vi "replaceBalanceToken.vi"(8 "error in (no error)":errorcluster, 10 "Query In":string, 11 "Banking Transaction in":refnum<class "Banking Transaction.lvclass">) -> (0 "error out":errorcluster, 2 "Query Out":string, 3 "Banking Transaction out":refnum<class "Banking Transaction.lvclass">)   [LabVIEW 2018, in "Banking Transaction.lvclass"]
uses:
  Banking Transaction.lvclass
  Banking Transaction.lvclass/Banking Transaction.ctl
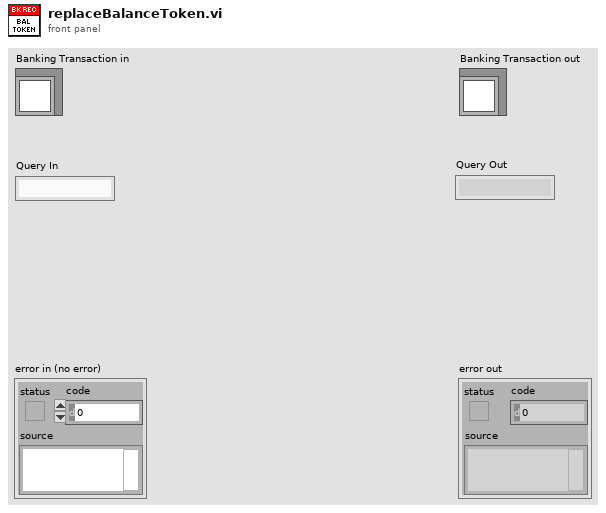
[diagram p1: front panel]
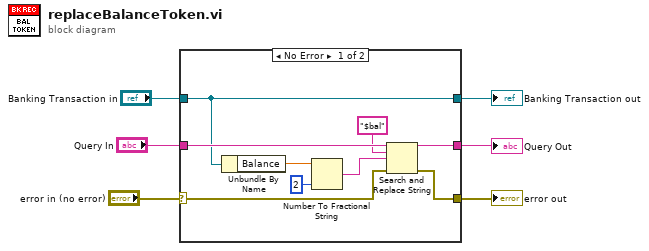
[diagram p0: block diagram]
diagram:
  n1 = case shown="No Error" "error in (no error)" {
    selector: "error in (no error)" -> [w12 w18]
    tunnel: "Query In" -> [w15 w17]
    tunnel: [w14 w17] -> w5
    tunnel: "Banking Transaction in" -> [w10 w16]
    tunnel: [w10 w16] -> w3
    tunnel: [w11 w18] -> w1
    frame No Error {
      n2 = Unbundle By Name(w10) -> ("Balance"=w9:dbl)
      n3 = Number To Fractional String(number=w9, precision (6)=i16 2) -> (F-format string=w8:string)  [unwired: 2 in]
      n4 = Search and Replace String(input string=w15, search string="$bal", replace string=w8, error in=w12) -> (result string=w14:string, error out=w11:errorcluster)  [unwired: 4 in, 2 out]
    }
    frame Error {
    }
  }
  "error out" <- w1
  "Banking Transaction out" <- w3
  "Query Out" <- w5
